vi "DSF.Engine.Plugin.Set Interface.vi"(10 "Interface":refnum<class "DSF.Engine.Interface.Plugin.lvclass">, 11 "Plugin in":refnum<class "DSF.Engine.Plugin.lvclass">) -> (3 "Plugin out":refnum<class "DSF.Engine.Plugin.lvclass">)   [LabVIEW 2017, in "DSF.Engine.lvlib" / "DSF.Engine.Plugin.lvclass"]
uses:
  DSF.Engine.Plugin.lvclass
  Interface/DSF.Engine.Interface.Plugin.lvclass
  DSF.Engine.Plugin.lvclass/DSF.Engine.Plugin.ctl
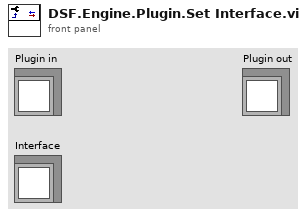
[diagram p1: front panel]
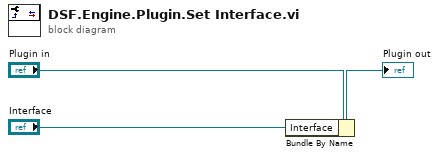
[diagram p0: block diagram]
diagram:
  n1 = Bundle By Name(cluster="Plugin in", "Interface"="Interface") -> (→"Plugin out":refnum<class "DSF.Engine.Plugin.lvclass">)
